vi "Y Axis Motor state control.vi"(11 "Y Axis Motor Target":T1) -> (3 "Y Axis Motor Params":T1)   [LabVIEW 2018]
panel:
  in  "stop":bool
  in  "error in (no error)":errorcluster
  out "error out":errorcluster
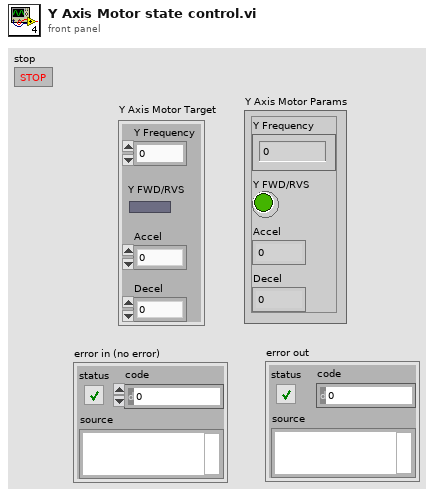
[diagram p1: front panel]
types:
  T1 = cluster{"Y Frequency":dbl, "Y FWD/RVS":bool, "Accel":dbl, "Decel":dbl}
  T2 = cluster{"Y Frequency":dbl, "Y FWD/RVS":bool, "Y Accel":dbl, "Y Decel":dbl}
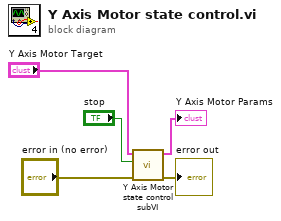
[diagram p0: block diagram]
diagram:
  n1 = call "Y Axis Motor state control subVI.vi"("error in (no error)"="error in (no error)", "stop"="stop", "Y Axis Motor Target"="Y Axis Motor Target") -> ("error out"=→"error out":errorcluster, "Y Axis Motor Params"=→"Y Axis Motor Params":T2)  [unwired: 7 in]
